vi "new records.vi"(7 "SA data":T1, 8 "Countries (in)":string[](array[string]), 9 "US data":T1, 10 "deaths CSV":string[][](array[string]), 11 "cases CSV":string[][](array[string])) -> ()   [LabVIEW 2019]
panel:
  out "record deaths":string[](array[string])
  out "record cases":string[](array[string])
  in  "Numeric Control":i32=-1
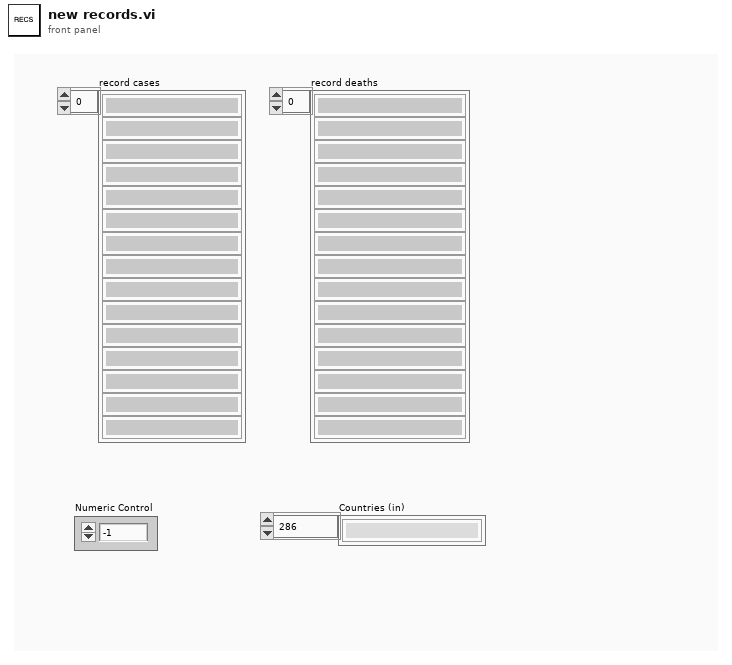
[diagram p1: front panel]
types:
  T1 = cluster{"cumulative deaths":i32[][], "deaths per day":i32[][], "case per day":i32[][], "cumulative cases":i32[][]}
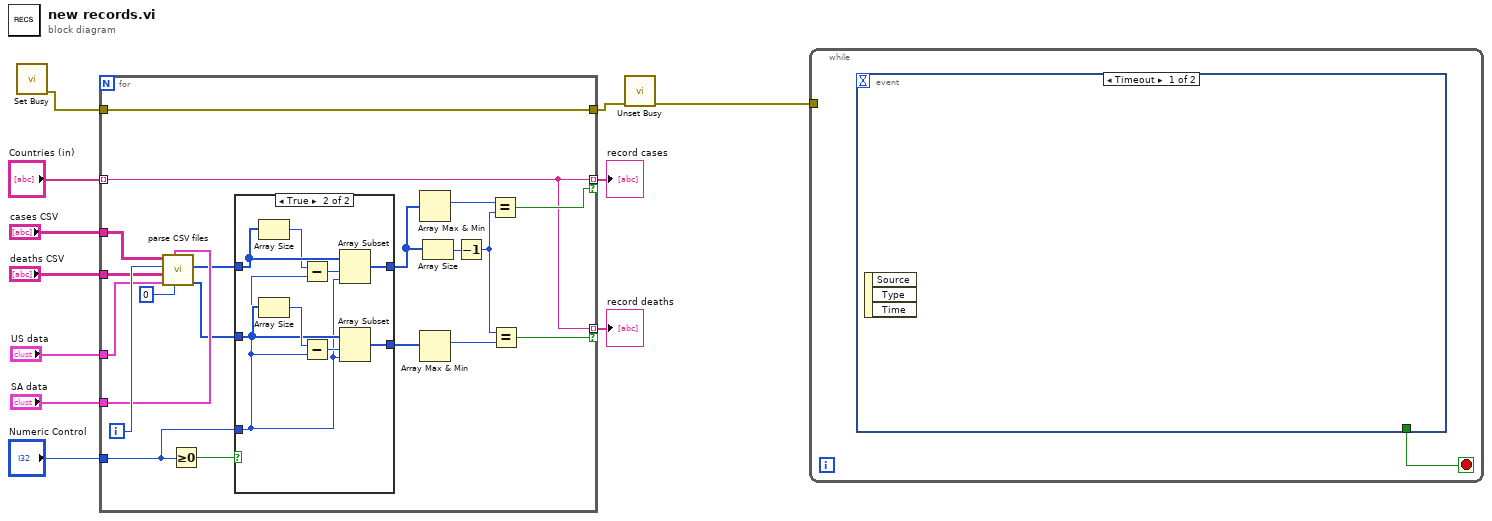
[diagram p0: block diagram]
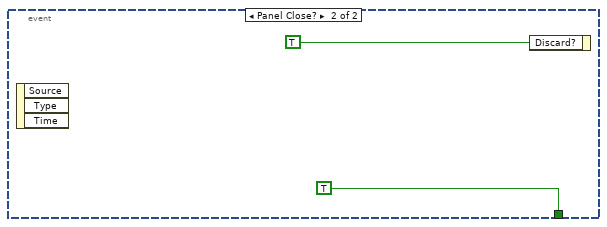
[diagram p3: hidden frame]
diagram:
  n1 = call <vilib>:"Set Busy.vi"() -> ("error out"=w4:errorcluster)  [unwired: 10 in, 1 out]
  n2 = for {
    tunnel: "Countries (in)" -> [w20] mode=indexing
    tunnel: "cases CSV" -> [w30]
    tunnel: "deaths CSV" -> [w29]
    tunnel: "US data" -> [w28]
    tunnel: "SA data" -> [w27]
    tunnel: [w20] -> w6 mode=indexing if=w21
    tunnel: [w20] -> w5 mode=indexing if=w19
    tunnel: w4 -> [w18]
    tunnel: [w18] -> w3
    tunnel: "Numeric Control" -> [w12]
    i -> [w31]
    n3 = call "parse CSV files.vi"("threshold cases"=u32 0, "SA data"=w27, "US data"=w28, "deaths CSV"=w29, "country index"=w31, "cases CSV"=w30) -> ("new deaths per day"=w15:i32[], "new cases per day"=w17:i32[])  [unwired: 4 out]
    n4 = Greater Or Equal To 0?(x=w12) -> (x >= 0?=w13:bool)
    n5 = case shown="True" w13 {
      tunnel: w17 -> [w33 w41]
      tunnel: [w33 w42] -> w16
      tunnel: w15 -> [w32 w35]
      tunnel: [w32 w36] -> w14
      tunnel: w12 -> [_ w34]
      frame False {
      }
      frame True {
        n6 = Array Size(array=w41) -> (size(s)=w39:i32)
        n7 = Array Size(array=w35) -> (size(s)=w38:i32)
        n8 = Subtract(x=w39, y=w34) -> (x-y=w40:i32)
        n9 = Subtract(x=w38, y=w34) -> (x-y=w37:i32)
        n10 = Array Subset(array=w41, index=w40, length=w34) -> (w42:i32[])
        n11 = Array Subset(array=w35, index=w37, length=w34) -> (w36:i32[])
      }
    }
    n12 = Array Max & Min(array=w16) -> (max index (indices)=w24:i32)  [unwired: 3 out]
    n13 = Array Max & Min(array=w14) -> (max index (indices)=w23:i32)  [unwired: 3 out]
    n14 = Array Size(array=w16) -> (size(s)=w25:i32)
    n15 = Decrement(x=w25) -> (x-1=w22:i32)
    n16 = Equal?(x=w24, y=w22) -> (x = y?=w21:bool)
    n17 = Equal?(x=w22, y=w23) -> (x = y?=w19:bool)
  }
  "record cases" <- w6
  "record deaths" <- w5
  n18 = call <vilib>:"Unset Busy.vi"("error in (no error)"=w3) -> ("error out"=w2:errorcluster)  [unwired: 10 in]
  n19 = while {
    tunnel: w2 -> [_]
    stop <- w43 stop-if-true
    n20 = event shown="[0] Timeout" {
      selector: _ -> [_ _]
      dyn-events: _ -> [_ _]
      timeout: _ -> [_ _]
      tunnel: [_ TRUE] -> w43
      event Timeout {
        n21 = event-data() -> ()  [unwired: 1 in, 3 out]
      }
      event Panel Close? {
        n22 = event-data() -> ()  [unwired: 1 in, 3 out]
        n23 = event-data("Discard?"=TRUE) -> ()  [unwired: 1 in, 1 out]
      }
    }
  }
